vi "joystick_read.vi"(0 "Refnum in":refnum<k1>, 5 "error in (no error)":errorcluster) -> (8 "X axis":i32, 9 "button 1":bool, 10 "pov 1":i32, 11 "button 2":bool, 12 "Z axis":i32, 13 "Y axis rotation":i32, 14 "Refnum out":refnum<k1>, 15 "button 3":bool, 16 "Y axis":i32, 17 "button 4":bool, 18 "X axis rotation":i32, 19 "error out":errorcluster)   [LabVIEW 2016]
uses:
  <vilib>/Utility/inputDevices.llb/joystickAcquire.vi
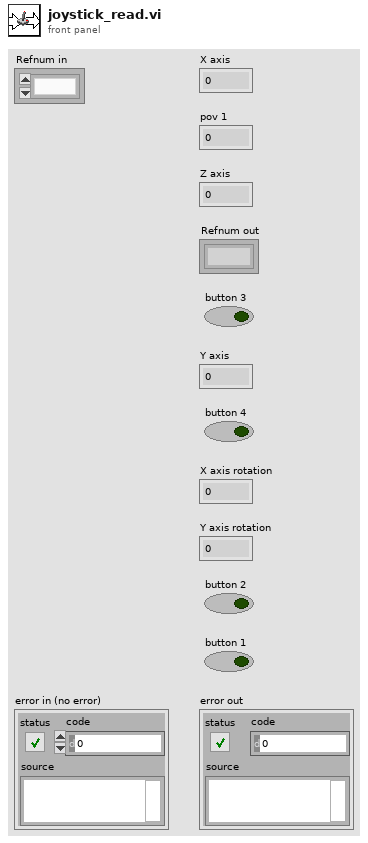
[diagram p1: front panel]
types:
  T1 = cluster{"X axis":i32, "Y axis":i32, "Z axis":i32, "X axis rotation":i32, "Y axis rotation":i32, "Z axis rotation":i32, "U axis":i32, "V axis":i32}
  T2 = cluster{"button 1":bool, "button 2":bool, "button 3":bool, "button 4":bool, "button 5":bool, "button 6":bool, "button 7":bool, "button 8":bool, "button 9":bool, "button 10":bool, "button 11":bool, "button 12":bool, "button 13":bool, "button 14":bool, "button 15":bool, "button 16":bool, "button 17":bool, "button 18":bool, "button 19":bool, "button 20":bool, "button 21":bool, "button 22":bool, "button 23":bool, "button 24":bool, "button 25":bool, "button 26":bool, "button 27":bool, "button 28":bool, "button 29":bool, "button 30":bool, "button 31":bool, "button 32":bool}
  T3 = cluster{"pov 1":i32, "pov 2":i32, "pov 3":i32, "pov 4":i32}
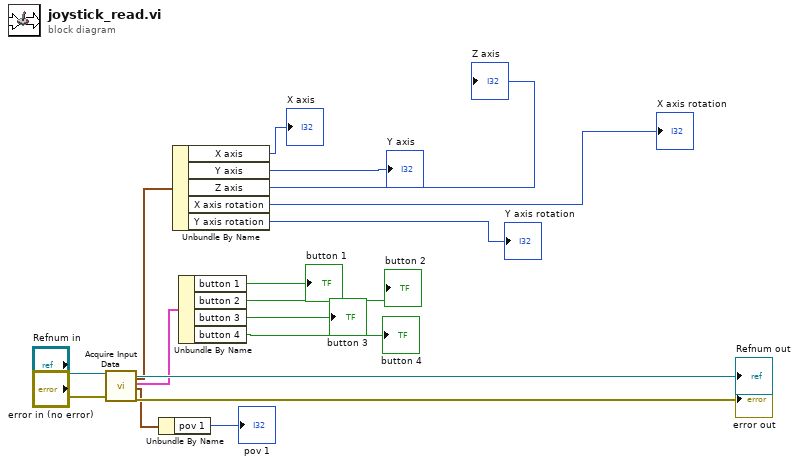
[diagram p0: block diagram]
diagram:
  n1 = call-poly <vilib>:"Acquire Input Data.vi"("device ID"="Refnum in", "error in (no error)"="error in (no error)") -> ("device ID"=→"Refnum out":refnum<k1>, "axis info"=w2:T1, "button info"=w3:T2, "direction info"=w4:T3, "error out"=→"error out":errorcluster)  [unwired: 13 in]
  n2 = Unbundle By Name(w4) -> ("pov 1"=→"pov 1":i32)
  n3 = Unbundle By Name(w2) -> ("X axis"=→"X axis":i32, "Y axis"=→"Y axis":i32, "Z axis"=→"Z axis":i32, "X axis rotation"=→"X axis rotation":i32, "Y axis rotation"=→"Y axis rotation":i32)
  n4 = Unbundle By Name(w3) -> ("button 1"=→"button 1":bool, "button 2"=→"button 2":bool, "button 3"=→"button 3":bool, "button 4"=→"button 4":bool)
